vi "RTC_Reading.vi"(2 "SRV In":string) -> (1 "Time (msec)":dbl, 4 "SRV Out":string="169.254.0.10")   [LabVIEW 2009]
panel:
  out "Reply":string
  # "This LabVIEW item is deprecated.\n\nIt is believed to be unused and will be removed in a future version of SRV."
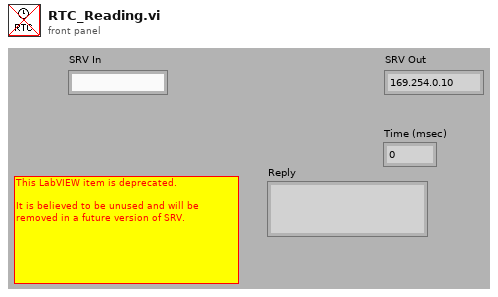
[diagram p1: front panel]
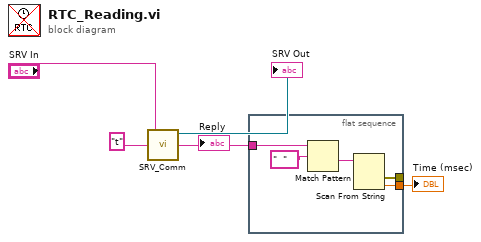
[diagram p0: block diagram]
diagram:
  n1 = call "SRV_Comm.vi"("Command Sent"="t", "SRV In"="SRV In") -> ("Reply"=w5:string, "SRV Out"=→"SRV Out":refnum<k5>)  [unwired: 1 in, 1 out]
  "Reply" <- w5
  n2 = flat-sequence {
    tunnel: w5 -> [w10]
    tunnel: [w9] -> w4
    tunnel: [w6] -> _
    frame #0 {
      n3 = Match Pattern(string=w10, regular expression="  " ("Command Sent")) -> (after substring=w8:string)  [unwired: 1 in, 3 out]
      n4 = Scan From String(input string=w8) -> (error out=w6:errorcluster, output 1=w9:dbl)  [unwired: 4 in, 2 out]
    }
  }
  "Time (msec)" <- w4
